vi "RT_Main.vi"() -> ()   [LabVIEW 2019]
uses:
  <vilib>/rvi/interface/nirviOpenFPGA/nirviOpenFPGA.xnode
  <vilib>/rvi/interface/nirviCloseFPGA/nirviCloseFPGA.xnode
  <vilib>/rvi/interface/nirviMethod/nirviMethod.xnode
  <vilib>/FPGAPlugInAG/Dynamic/niLvFpga_Run_Dynamic.vi
  <vilib>/FPGAPlugInAG/Dynamic/niLvFpga_Abort_Dynamic.vi
  <vilib>/rvi/interface/nirviReadWriteControl/nirviReadWriteControl.xnode
  <vilib>/Platform/TimedLoop/XDataNode/wakeup.ctl
  <vilib>/Platform/TimedLoop/XDataNode/XDNodeRunTimeDep.lvlib
  <vilib>/Platform/TimedLoop/XDataNode/nitl_modes.ctl
  <vilib>/Platform/TimedLoop/XDataNode/timing_clust.ctl
  <vilib>/platform/TimedLoop/XDataNode/XDataNode.xnode
  FPGA Bitfiles/hipexov3fpga_FPGATarget_Main_w1sytSUJKDk.lvbitx
  FPGA_Main.vi
  <vilib>/FPGAPlugInAG/myRIO-1900/niLvFpga_Open_myRIO-1900.vi
  <vilib>/rvi/interface/common/dynamic/niFpgaDynamicAddResources.vi
  NiFpgaLv.dll
  <vilib>/Utility/error.llb/Error Cluster From Error Code.vi
  <vilib>/rvi/interface/Simulation/niFpgaSimulationCallBeginRW.vi
  <vilib>/rvi/errors/niLvFpgaAdjustHostInterfaceError.vi
  <vilib>/FPGAPlugInAG/Dynamic/niLvFpga_Close_Dynamic.vi
panel:
  out "Desired Frequency":dbl
  in  "increment freq":bool
  in  "Saving File Name":string
  out "TOR MEA":cluster{dbl, dbl}(graph)
  in  "SINE?":bool
  in  "Torque Set":dbl
  out "Current Des":dbl(graph)
  out "RT RATE (MS)":u32
  in  "stop":bool
  in  "ASSIST":bool
  in  "L_TRQ_DES":fxp<+/-,32,16>
  in  "ENC INIT":bool
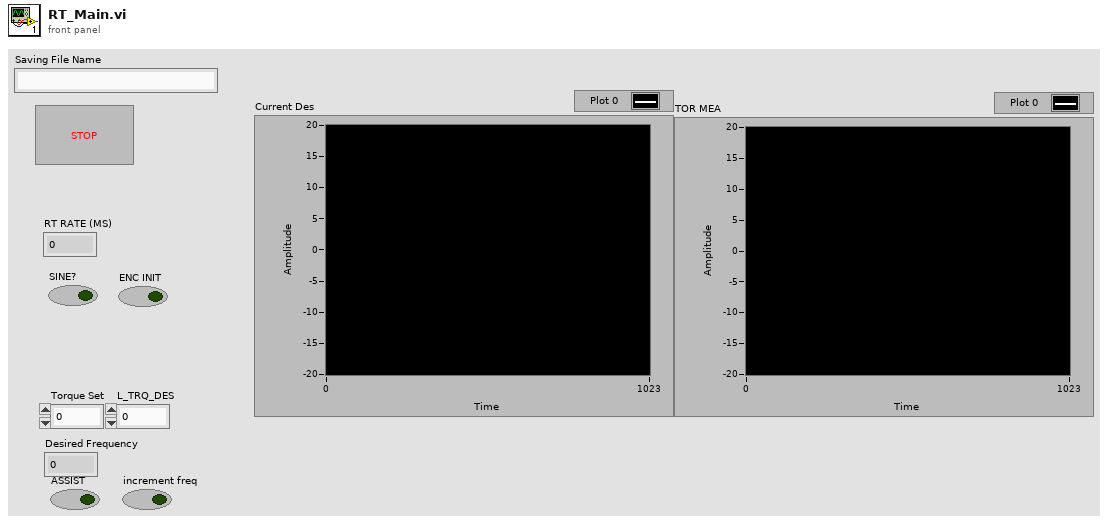
[diagram p1: front panel]
types:
  T1 = enum16{"open", "replace", "create", "open or create", "replace or create", "replace or create with confirmation"}
  T2 = typedef "XDNodeRunTimeDep.lvlib/timing_clust.ctl" = cluster{"Expected End [f-1]":u64, "Actual End [f-1]":u64, "Finished Late? [f-1]":bool, "Expected End [i-1]":u64, "Actual End [i-1]":u64, "Finished Late? [i-1]":bool, "Expected Start [i]":u64, "Actual Start [i]":u64, "Expected Start [f]":u64, "Actual Start [f]":u64, "Source Name":string, "Structure Name":string, "Period":i64, "Deadline":i64, "Offset":i64, "Start":i64, "Priority":i32, "Timeout":i32, "Mode":T3, "Wakeup Reason":T4, "Error":errorcluster, "Source Type":string, "Secondary Source Type":string, "Global End Time":u64, "Global Start Time":u64, "Frame Duration":u64, "Iteration Duration":u64, "Assigned CPU":i32, "I/O Scan Engine Mode":u32}
  T3 = typedef "XDNodeRunTimeDep.lvlib/nitl_modes.ctl" = enum32{"No Change", "Process missed periods, maintain original phase", "Discard missed periods, maintain original phase", "Process missed periods, ignore original phase", "Discard missed periods, ignore original phase"}
  T4 = typedef "XDNodeRunTimeDep.lvlib/wakeup.ctl" = enum32{"Normal", "Aborted", "Asynchronous wakeup", "Timing source error", "Timed loop error", "Timeout"}
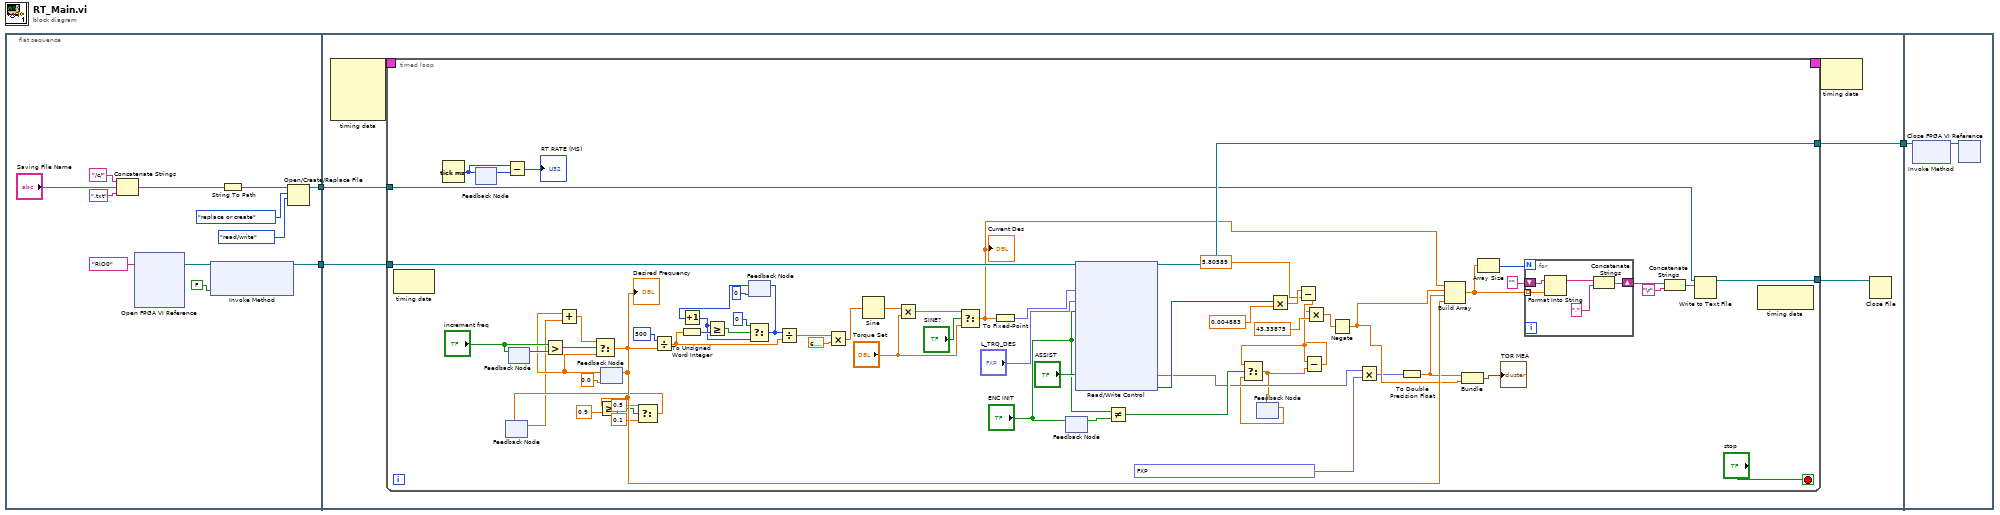
[diagram p0: block diagram]
diagram:
  n1 = flat-sequence {
    tunnel: [w13] -> w3
    tunnel: [w4] -> w1
    tunnel: w3 -> [w19]
    tunnel: [w18] -> w2
    tunnel: w1 -> [w17]
    tunnel: w2 -> [w97]
    frame #0 {
      n2 = Concatenate Strings("/c/" ("string"), "Saving File Name", ".txt" ("string")) -> (w11:string)
      n3 = xnode "Open FPGA VI Reference"("resource name"=tag "RIO0") -> ("FPGA VI Reference Out"=w14:refnum<k20>)  [unwired: 1 in, 1 out]
      n4 = xnode "Invoke Method"("FPGA VI Reference In"=w14, "Wait Until Done (F)"=FALSE) -> ("FPGA VI Reference Out"=w13:refnum<k20>)  [unwired: 1 in, 1 out]
      n5 = String To Path(string=w11) -> (path=w7:path)
      n6 = Open/Create/Replace File(file path (use dialog)=w7, operation (0:open)=T1."replace or create", access (0:read/write)=enum16{"read/write", "read-only", "write-only"}."read/write") -> (refnum out=w4:refnum<file>)  [unwired: 3 in, 2 out]
    }
    frame #1 {
      n7 = node-c288() -> (w21:T2)  [unwired: 4 in]
      n8 = timed-loop {
        tunnel: w19 -> [w86]
        tunnel: [w85] -> w18
        timing: w21 -> [_]
        timing-out: [_] -> w20
        tunnel: w17 -> [w54]
        tunnel: [w53] -> w16
        stop <- "stop" stop-if-true
        n9 = node-c288() -> ()  [unwired: 1 in, 1 out]
        n10 = Tick Count (ms)() -> (millisecond timer value=w80:u32)
        n11 = feedback-in #1(w80) -> ()
        n12 = feedback #1() -> (w81:u32)  [unwired: 1 in]
        n13 = feedback #2() -> (w36:dbl)  [unwired: 1 in]
        n14 = Subtract(x=w80, y=w81) -> (x-y=→"RT RATE (MS)":u32)
        n15 = feedback-in #3("increment freq") -> ()
        n16 = feedback #3() -> (w52:bool)  [unwired: 1 in]
        n17 = Greater?(x="increment freq", y=w52) -> (0:w50:bool)
        n18 = feedback #4(0.0) -> (w49:dbl)
        n19 = Add(x=w49, y=w36) -> (x+y=w48:dbl)
        n20 = Select(t=w48, s=w50, f=w49) -> (s? t:f=w42:dbl)
        "Desired Frequency" <- w42
        n21 = Greater Or Equal?(x=w42, y=0.9) -> (x >= y?=w40:bool)
        n22 = feedback-in #4(w42) -> ()
        n23 = Select(t=0.5, s=w40, f=0.1) -> (s? t:f=w37:dbl)
        n24 = feedback-in #2(w37) -> ()
        n25 = Divide(x=500, y=w42) -> (x/y=w70:dbl)
        n26 = To Unsigned Word Integer(number=w70) -> (unsigned 16bit integer=w77:u16)
        n27 = feedback #5(0) -> (w73:i32)
        n28 = Increment(x=w73) -> (x+1=w74:i32)
        n29 = Greater Or Equal?(x=w74, y=w77) -> (x >= y?=w76:bool)
        n30 = Select(t=0, s=w76, f=w74) -> (s? t:f=w71:i32)
        n31 = feedback-in #5(w71) -> ()
        n32 = Divide(x=w71, y=w70) -> (x/y=w69:dbl)
        n33 = Multiply(x=w69, y=6.283185307179586) -> (x*y=w67:dbl)
        n34 = Sine(x=w67) -> (sin(x)=w66:dbl)
        n35 = Multiply(x=w66, y="Torque Set") -> (x*y=w61:dbl)
        n36 = Select(t=w61, s="SINE?", f="Torque Set") -> (s? t:f=w46:dbl)
        "Current Des" <- w46
        n37 = To Fixed-Point(number=w46) -> (fixed-point=w64:fxp<+/-,32,16>)  [unwired: 1 in]
        n38 = feedback #6() -> (w45:bool)  [unwired: 1 in]
        n39 = feedback-in #6("ENC INIT") -> ()
        n40 = xnode "Read/Write Control"("FPGA VI Reference In"=w86, "R_TRQ_DES"=w64, "L_TRQ_DES"="L_TRQ_DES", "ENC INIT"="ENC INIT", "ASSIST"="ASSIST") -> ("FPGA VI Reference Out"=w85:refnum<k20>, "R SPRING TORQUE"=w28:fxp<+/-,64,24>, "FUTEK"=w63:i16)  [unwired: 1 in, 6 out]
        n41 = Not Equal?(x="ENC INIT", y=w45) -> (x != y?=w43:bool)
        n42 = feedback #7() -> (w25:dbl)  [unwired: 1 in]
        n43 = Multiply(x=w63, y=0.004883) -> (x*y=w31:dbl)
        n44 = Subtract(x=w31, y=5.80589 ("Voltage Offset")) -> (x-y=w23:dbl)
        n45 = Select(t=w23, s=w43, f=w25) -> (s? t:f=w24:dbl)
        n46 = feedback-in #7(w24) -> ()
        n47 = Subtract(x=w23, y=w24) -> (x-y=w22:dbl)
        n48 = Multiply(x=w22, y=43.33875) -> (x*y=w30:dbl)
        n49 = Negate(x=w30) -> (-x=w29:dbl)
        n50 = Multiply(x=w28, y=fxp<+/-,53,13> 1.2200000000002547) -> (x*y=w27:fxp<+/-,64,36>)
        n51 = To Double Precision Float(number=w27) -> (double precision float=w34:dbl)
        n52 = Build Array(w46, w29, w34, w42) -> (w60:dbl[])
        n53 = Bundle(w34, w29) -> (→"TOR MEA":cluster{dbl, dbl})  [unwired: 1 in]
        n54 = Array Size(array=w60) -> (size(s)=w59:i32)
        n55 = for {
          N: w59 -> [_]
          tunnel: w60 -> [w92] mode=indexing
          shift-right: [w89] -> w57
          shift-left: "" -> [w88]
          n56 = Format Into String(initial string=w88, w92) -> (resulting string=w91:string)  [unwired: 2 in, 1 out]
          n57 = Concatenate Strings(w91, "," ("string")) -> (w89:string)
        }
        n58 = Concatenate Strings(w57, "\r") -> (w55:string)
        n59 = Write to Text File(file (use dialog)=w54, text=w55) -> (refnum out=w53:refnum<file>)  [unwired: 2 in, 2 out]
        n60 = node-c288() -> ()  [unwired: 1 in, 1 out]
      }
      n61 = node-c288(w20) -> ()  [unwired: 1 out]
      n62 = Close File(refnum=w16) -> ()  [unwired: 1 in, 2 out]
    }
    frame #2 {
      n63 = xnode "Invoke Method"("FPGA VI Reference In"=w97) -> ("FPGA VI Reference Out"=w98:refnum<k20>)  [unwired: 1 in, 1 out]
      n64 = xnode "Close FPGA VI Reference"("FPGA VI Reference In"=w98) -> ()  [unwired: 1 in, 1 out]
    }
  }
